vi "NativeTypesTester.vi"() -> ()   [LabVIEW 2013]
doc: "Tester for the NativeTypes API"
uses:
  FA_DeviceConfig.ctl
  FA_Config.ctl
  FA_LocalStore API/source/VI Source/FA_LSSpecialTypes.ctl
  FA_ConfigItem.ctl
  FA_NativeTypes.lvlib
  FA_LocalStore API/source/VI Source/FA_LocalStore.lvlib
panel:
  out "DeviceConfig 2":T1
  out "ConfigData":T2
  out "Items 2":T4
  in  "Items":T4={"Item"=[{"Name"="myName", "ConfigId"="myConfigID", "ModificationDate"="myDate0", "ETag"="myETag"}, {"Name"="myName1", "ConfigId"="myConfigID1", "ModificationDate"="myDate1", "ETag"="myETag1"}]}
  in  "Configuration":T2={"Id"="e3849b4f-2e91-4de2-ac11-d7b5db970655", "Name"="RTEXE", "Parameter"=[{"Name"="parameter0", "Value"="value2"}, {"Name"="parameter1", "Value"="value1"}], "Account"="0000", "CreateDate"="2012-07-13T20:14:27.770Z", "LastModified"="2012-07-13T20:14:27.815Z"}
  in  "DeviceConfig":T1={"DeviceId"="device1", "Account"="5678", "DeviceConfigEntry"=[{"ConfigId"="0dac3609-a663-42f1-bc0b-7e1790b8cb89", "Purpose"="main-configuration"}], "Parameter"=[{"Name"="parameter2", "Value"="value3"}, {"Name"="parameter1", "Value"="value1"}], "CreateDate"="2012-06-04T21:43:55.372Z", "LastModified"="2012-06-14T18:52:33.664Z"}
  out "Error Out":errorcluster
  in  "Error In":errorcluster
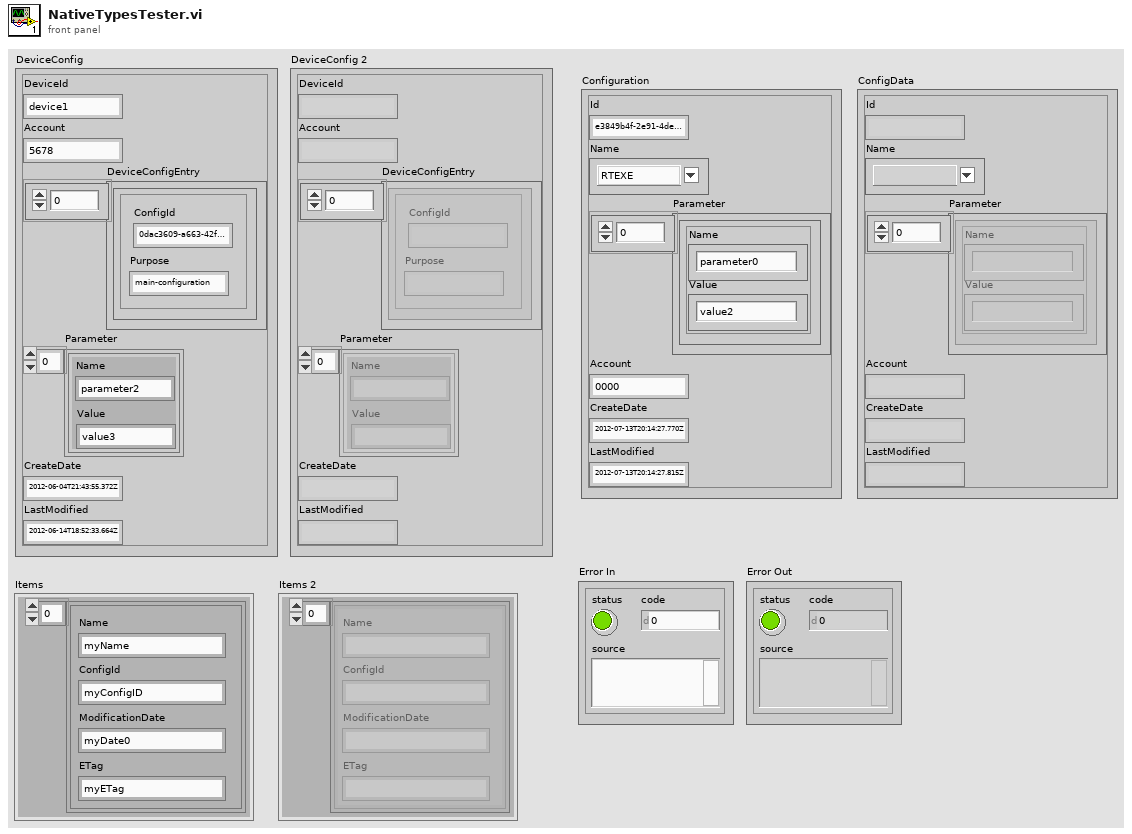
[diagram p1: front panel]
types:
  T1 = typedef "FA_NativeTypes.lvlib/FA_DeviceConfig.ctl" = cluster{"DeviceId":string, "Account":string, "DeviceConfigEntry":cluster{"ConfigId":string, "Purpose":string}[], "Parameter":cluster{"Name":string, "Value":string}[], "CreateDate":string, "LastModified":string}
  T2 = typedef "FA_NativeTypes.lvlib/FA_Config.ctl" = cluster{"Id":string, "Name":T3, "Parameter":cluster{"Name":string, "Value":string}[], "Account":string, "CreateDate":string, "LastModified":string}
  T3 = typedef "FA_LocalStore.lvlib/FA_LSSpecialTypes.ctl" = string
  T4 = typedef "FA_NativeTypes.lvlib/FA_ConfigItem.ctl" = cluster{"Item":cluster{"Name":string, "ConfigId":string, "ModificationDate":string, "ETag":string}[]}
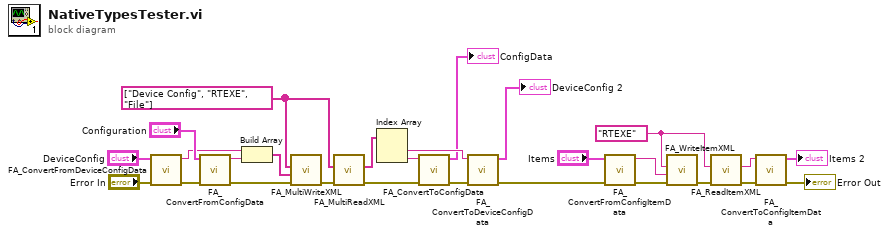
[diagram p0: block diagram]
diagram:
  w5 = T3 "RTEXE" ("Special Type")
  w18 = T3[] ["Device Config", "RTEXE", "File"] ("Special Type Array")
  n1 = call "FA_ConvertFromDeviceConfigData.vi"("Error In"="Error In", "DeviceConfig"="DeviceConfig") -> ("Error Out"=w26:errorcluster, "XML String"=w22:string)  [unwired: 8 in]
  n2 = call "FA_ConvertFromConfigData.vi"("Error In"=w26, "Config"="Configuration") -> ("Error Out"=w9:errorcluster, "XML String"=w21:string)  [unwired: 8 in]
  n3 = Build Array(w22, w21) -> (w20:string[])
  n4 = call "FA_MultiWriteXML.vi"("Error In"=w9, "XML String Array"=w20, "Special Type Array"=w18) -> ("Error Out"=w19:errorcluster)  [unwired: 6 in]
  n5 = call "FA_MultiReadXML.vi"("Error In"=w19, "Special Type Array"=w18) -> ("Error Out"=w10:errorcluster, "XML String Array"=w17:string[])  [unwired: 6 in]
  n6 = Index Array(array=w17) -> (element #1=w16:string, element #2=w15:string)  [unwired: 2 in]
  n7 = call "FA_ConvertToConfigData.vi"("Error In"=w10, "XML String"=w15) -> ("Error Out"=w14:errorcluster, "ConfigData"=→"ConfigData":T2)  [unwired: 8 in]
  n8 = call "FA_ConvertToDeviceConfigData.vi"("Error In"=w14, "XML String"=w16) -> ("Error Out"=w8:errorcluster, "DeviceConfig"=→"DeviceConfig 2":T1)  [unwired: 8 in]
  n9 = call "FA_ConvertFromConfigItemData.vi"("Error In"=w8, "Items"="Items") -> ("Error Out"=w1:errorcluster, "XML String"=w7:string)  [unwired: 8 in]
  n10 = call "FA_WriteItemXML.vi"("Error In"=w1, "XML String"=w7, "Special Type"=w5) -> ("Error Out"=w6:errorcluster)  [unwired: 6 in]
  n11 = call "FA_ReadItemXML.vi"("Error In"=w6, "Special Type"=w5) -> ("Error Out"=w4:errorcluster, "XML String"=w3:string)  [unwired: 6 in]
  n12 = call "FA_ConvertToConfigItemData.vi"("Error In"=w4, "XML String"=w3) -> ("Error Out"=→"Error Out":errorcluster, "Items"=→"Items 2":T4)  [unwired: 8 in]
